vi "TonePattern-Create.vi"(0 "Data in":T1, 9 "Npts":i32, 11 "error in (no error)":errorcluster) -> (4 "Data out":T1, 8 "Y":dbl[](array[numeric]), 15 "error out":errorcluster)   [LabVIEW 2020]
uses:
  TonePattern-Data.ctl
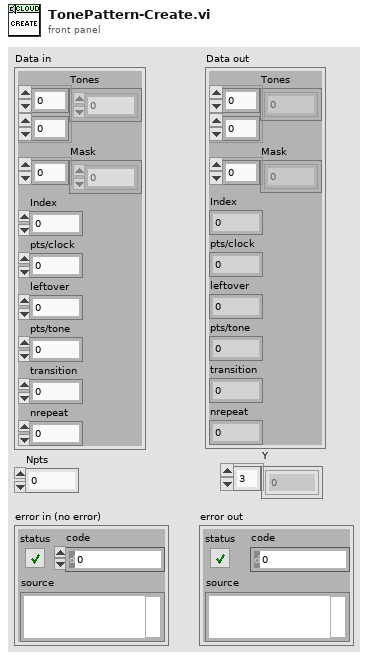
[diagram p1: front panel]
types:
  T1 = typedef "TonePattern-Data.ctl" = cluster{"Tones":dbl[][], "Mask":i32[], "Index":i32, "pts/clock":i32, "leftover":i32, "pts/tone":i32, "transition":i32, "nrepeat":i32}
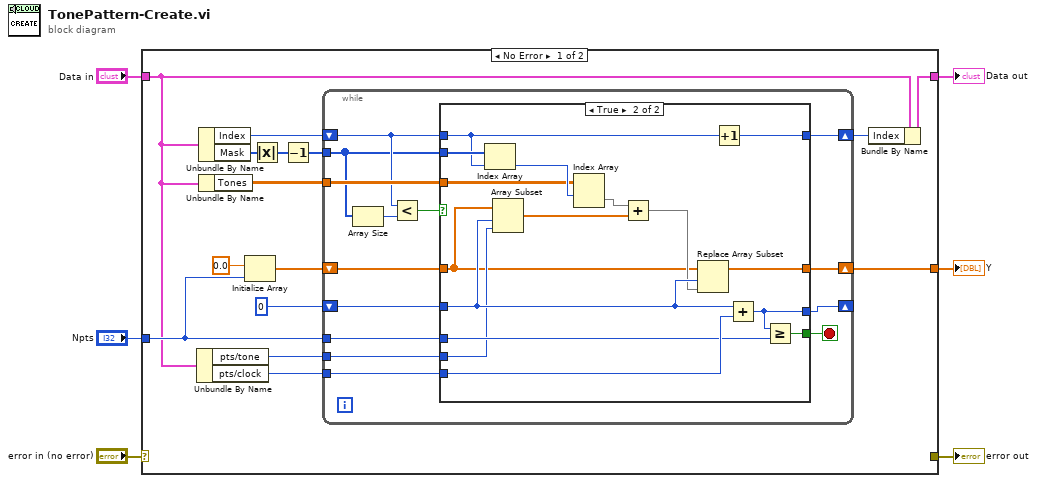
[diagram p0: block diagram]
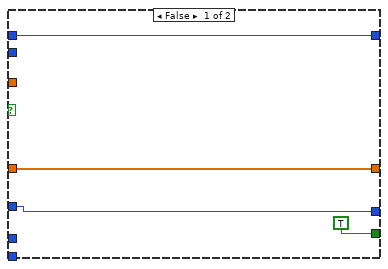
[diagram p2: hidden frame]
diagram:
  n1 = case shown="No Error" "error in (no error)" {
    selector: "error in (no error)" -> [_ w57]
    tunnel: "Data in" -> [w10 w56]
    tunnel: [w12 w56] -> w4
    tunnel: [_ w57] -> w5
    tunnel: "Npts" -> [w15 _]
    tunnel: [w18 _] -> w1
    frame No Error {
      n2 = Unbundle By Name(w10) -> ("pts/tone"=w14:i32, "pts/clock"=w16:i32)
      n3 = Unbundle By Name(w10) -> ("Index"=w13:i32, "Mask"=w19:i32[])
      n4 = Unbundle By Name(w10) -> ("Tones"=w9:dbl[][])
      n5 = Initialize Array(0.0, w15) -> (w20:dbl[])
      n6 = Absolute Value(x=w19) -> (abs(x)=w8:i32[])
      n7 = Decrement(x=w8) -> (x-1=w7:i32[])
      n8 = while {
        shift-right: [w33] -> w18
        shift-left: w20 -> [w34]
        tunnel: w7 -> [w23]
        tunnel: w9 -> [w35]
        shift-right: [w30] -> _
        shift-left: 0 -> [w32]
        tunnel: w16 -> [w31]
        tunnel: w15 -> [w29]
        tunnel: w14 -> [w27]
        shift-right: [w26] -> w11
        shift-left: w13 -> [w24]
        stop <- w28 stop-if-true
        n9 = Array Size(array=w23) -> (size(s)=w22:i32)
        n10 = Less?(x=w24, y=w22) -> (x < y?=w25:bool)
        n11 = case shown="True" w25 {
          tunnel: w23 -> [_ w55]
          tunnel: w35 -> [_ w53]
          tunnel: w34 -> [w38 w41]
          tunnel: [w38 w52] -> w33
          tunnel: w32 -> [w39 w50]
          tunnel: w31 -> [_ w48]
          tunnel: [w39 w47] -> w30
          tunnel: w29 -> [_ w46]
          tunnel: [TRUE w45] -> w28
          tunnel: w27 -> [_ w44]
          tunnel: w24 -> [w36 w43]
          tunnel: [w36 w42] -> w26
          frame False {
          }
          frame True {
            n12 = Index Array(array=w55, index=w43) -> (element=w54:i32)
            n13 = Array Subset(array=w41, index=w50, length=w44) -> (w51:dbl[])
            n14 = Index Array(array=w53, index (row)=w54) -> (element=w40:dbl[])  [unwired: 1 in]
            n15 = Add(x=w40, y=w51) -> (x+y=w49:dbl[])
            n16 = Replace Array Subset(array=w41, new element=w49, index=w50) -> (w52:dbl[])
            n17 = Increment(x=w43) -> (x+1=w42:i32)
            n18 = Add(x=w50, y=w48) -> (x+y=w47:i32)
            n19 = Greater Or Equal?(x=w47, y=w46) -> (x >= y?=w45:bool)
          }
        }
      }
      n20 = Bundle By Name(cluster=w10, "Index"=w11) -> (w12:T1)
    }
    frame Error {
    }
  }
  "error out" <- w5
  "Data out" <- w4
  "Y" <- w1
